vi "ErrorHandling.getLastNErrors.vi"(8 "error in (no error)":errorcluster, 10 "N":u32, 11 "ErrorHandling in":refnum<data-value>) -> (0 "error out":errorcluster, 2 "Errors":T1[](array[typedef]), 3 "ErrorHandling out":refnum<data-value>)   [LabVIEW 2016, in "ErrorHandling.lvclass"]
doc: "Gibt die letzten N Fehler aus\n\n17.04.14 / sige"
uses:
  ErrorHandling.lvclass
  ErrorHandling.OccurredErrorDataStruct.ctl
  ErrorHandling.lvclass/ErrorHandling.ctl
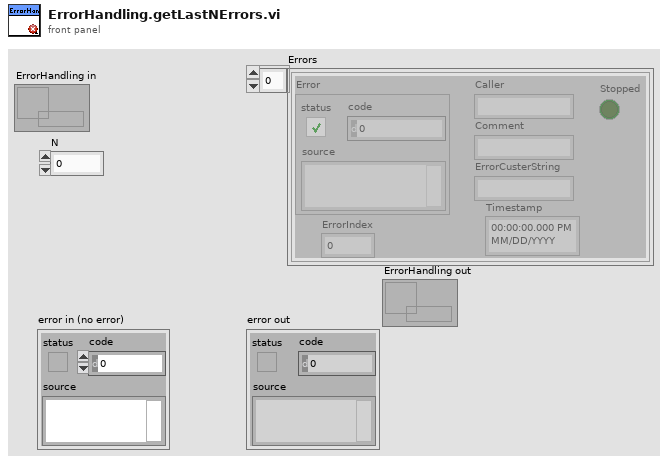
[diagram p1: front panel]
types:
  T1 = typedef "ErrorHandling.lvclass/ErrorHandling.OccurredErrorDataStruct.ctl" = cluster{"Error":errorcluster, "Caller":string, "Comment":string, "Timestamp":timestamp, "Stopped":bool, "ErrorCusterString":string, "ErrorIndex":u64}
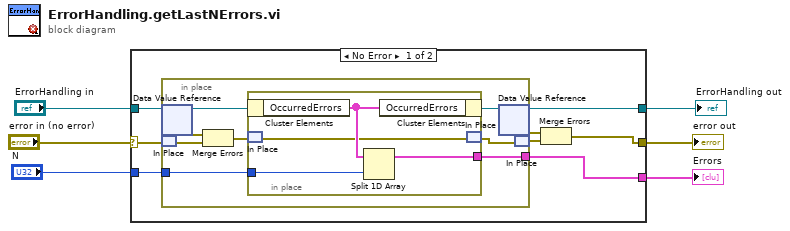
[diagram p0: block diagram]
diagram:
  n1 = case shown="No Error" "error in (no error)" {
    selector: "error in (no error)" -> [w10 w28]
    tunnel: [w7 w28] -> w5
    tunnel: [w11 w27] -> w1
    tunnel: "ErrorHandling in" -> [w12 w27]
    tunnel: "N" -> [w14 _]
    tunnel: [w13 _] -> w3
    frame No Error {
      n2 = in-place {
        in-place-border: w14 -> [w22]
        in-place-border: [w21] -> w13
        n3 = in-place-dvr #1(w12) -> (w20:refnum<class "ErrorHandling.lvclass">, w18:errorcluster)
        n4 = in-place-match #2(w10) -> (w15:errorcluster)
        n5 = Merge Errors(w18, w15) -> (w17:errorcluster)
        n6 = in-place {
          in-place-border: w22 -> [w26]
          in-place-border: [w25] -> w21
          n7 = in-place-cluster #3(w20) -> ("OccurredErrors"=w24:T1[])
          n8 = in-place-match #4(w17) -> (w23:errorcluster)
          n9 = Split 1D Array(array=w24, index=w26) -> (first subarray=w25:T1[])  [unwired: 1 out]
          n10 = in-place-cluster #3("OccurredErrors"=w24) -> (w19:refnum<class "ErrorHandling.lvclass">)
          n11 = in-place-match #4(w23) -> (w16:errorcluster)
        }
        n12 = in-place-dvr #1(w19) -> (w11:refnum<data-value>, w9:errorcluster)
        n13 = in-place-match #2(w16) -> (w8:errorcluster)
      }
      n14 = Merge Errors(w9, w8) -> (w7:errorcluster)
    }
    frame Error {
    }
  }
  "error out" <- w5
  "Errors" <- w3
  "ErrorHandling out" <- w1
